vi "Get Background Image JPG Name.vi"(3 "Inkscape Path":path) -> (1 "Background JPG Name":string)   [LabVIEW 2019]
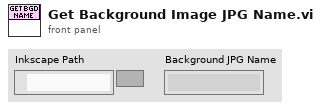
[diagram p1: front panel]
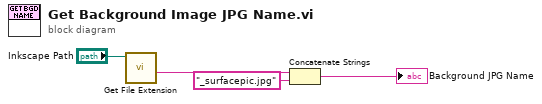
[diagram p0: block diagram]
diagram:
  n1 = call <vilib>:"Get File Extension.vi"("file"="Inkscape Path") -> ("filename without extension"=w4:string)  [unwired: 6 in, 4 out]
  n2 = Concatenate Strings(w4, "_surfacepic.jpg" ("string")) -> (→"Background JPG Name":string)
